vi "trad ligne lettre to chiffre.vi"(10 "face in":string[](array[string])=["w6", "w3", "w0", "b7", "b4", "b1", "b8", "b5", "b2"]) -> (2 "face  out":string[](array[string])=["w6", "w3", "w0", "b7", "b4", "b1", "b8", "b5", "b2"])   [LabVIEW 2019]
uses:
  <vilib>/regexp/Match Regular Expression.xnode
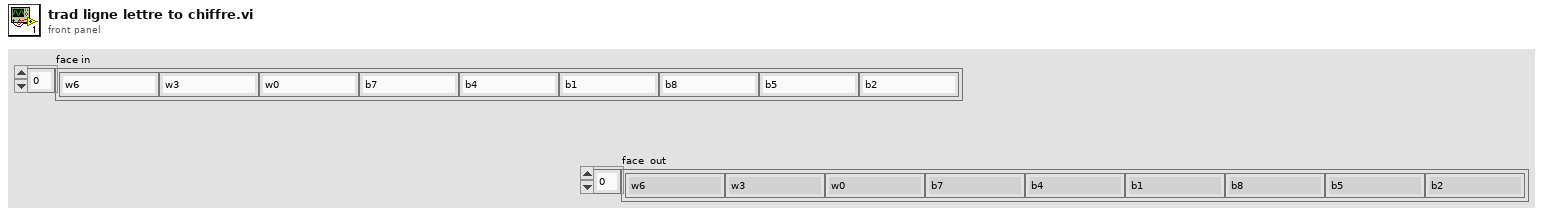
[diagram p1: front panel]
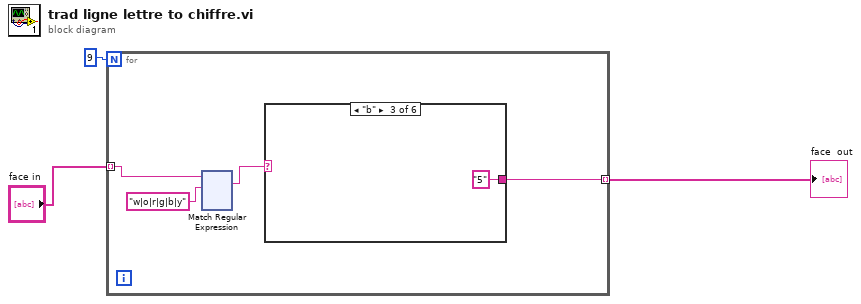
[diagram p0: block diagram]
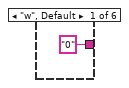
[diagram p2: hidden frame]
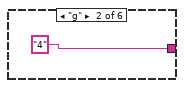
[diagram p3: hidden frame]
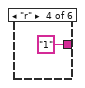
[diagram p4: hidden frame]
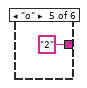
[diagram p5: hidden frame]
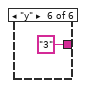
[diagram p6: hidden frame]
diagram:
  n1 = for {
    N: 9 -> [_]
    tunnel: "face in" -> [w6] mode=indexing
    tunnel: [w7] -> w1 mode=indexing
    n2 = xnode "Match Regular Expression"("input string"=w6, "regular expression"="w|o|r|g|b|y" ("input string")) -> ("whole match"=w4:string)  [unwired: 4 in, 4 out]
    n3 = case shown="\"b\"" w4 {
      tunnel: ["0" "4" "5" "1" "2" "3"] -> w7
      frame "w", Default {
      }
      frame "g" {
      }
      frame "b" {
      }
      frame "r" {
      }
      frame "o" {
      }
      frame "y" {
      }
    }
  }
  "face  out" <- w1
